vi "Test_InverseLogic_WriteZero_TerminalVisible.vi"(8 "error in (no error)":errorcluster, 11 "TestCase in":refnum<class "TestTerminalEnabledStateBinding.lvclass">) -> (0 "error out":errorcluster, 3 "TestCase out":refnum<class "TestTerminalEnabledStateBinding.lvclass">)   [LabVIEW 2017, in "TestTerminalEnabledStateBinding.lvclass"]
uses:
  TestTerminalEnabledStateBinding.lvclass
  Source/Concrete/TerminalEnabledStateBinding/TerminalEnabledStateBinding.lvclass
  C:/Git/composed-transport/Source/ITransport/ITransport.lvclass
  Source/ITransport/ITransport.lvclass
panel:
  in  "Numeric":i32
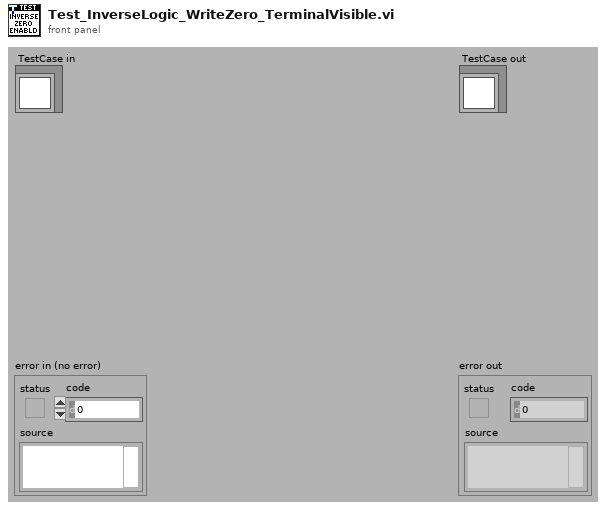
[diagram p1: front panel]
types:
  T1 = enum8{"Enabled", "Disabled", "Disabled and Grayed Out"}
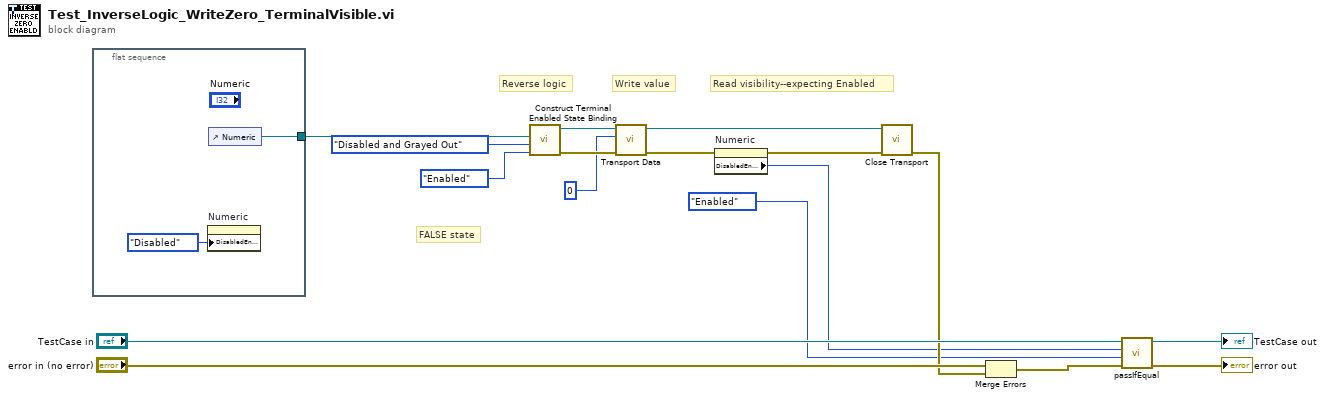
[diagram p0: block diagram]
diagram:
  # "FALSE state"
  # "Reverse logic"
  # "Read visibility--expecting Enabled"
  # "Write value"
  n1 = flat-sequence {
    tunnel: [w19] -> w9
    frame #0 {
      n2 = property on="Numeric" class="DigNum (strict)"("DisabledEnum"=T1."Disabled" ("Disabled")) -> ()  [unwired: 2 in, 2 out]
      n3 = control-ref of="Numeric"() -> (w19:refnum<vi>)
    }
  }
  n4 = call "Construct Terminal Enabled State Binding.vi"("FALSE State (Disabled and Grayed Out)"=T1."Enabled", "TRUE State (Enabled)"=T1."Disabled and Grayed Out", "Control"=w9) -> ("error out"=w11:errorcluster, "TerminalEnabledStateBinding"=w13:refnum<class "TerminalEnabledStateBinding.lvclass">)  [unwired: 7 in]
  n5 = call "Transport Data.vi"("error in (no error)"=w11, "Value"=0, "ITransport in"=w13) -> ("error out"=w8:errorcluster, "ITransport out"=w10:refnum<class "TerminalEnabledStateBinding.lvclass">)  [unwired: 7 in]
  n6 = property on="Numeric" class="DigNum (strict)"(error in=w8) -> (error out=w7:errorcluster, "DisabledEnum"=w3:T1)  [unwired: 1 in, 1 out]
  n7 = call-dynamic "Close Transport.vi"("error in (no error)"=w7, "ITransport in"=w10) -> ("error out"=w6:errorcluster)  [unwired: 9 in]
  n8 = Merge Errors("error in (no error)", w6) -> (w12:errorcluster)
  n9 = call-dynamic "passIfEqual.vi"("error in (no error)"=w12, "y"=T1."Enabled" ("FALSE State (Disabled and Grayed Out)"), "x"=w3, "TestCase in"="TestCase in") -> ("error out"=→"error out":errorcluster, "TestCase out"=→"TestCase out":refnum<class "TestTerminalEnabledStateBinding.lvclass">)  [unwired: 6 in]
